vi "Copy InstrumentStudio Template.vi"(8 "error in":errorcluster) -> (0 "error out":errorcluster)   [LabVIEW 2021, in "Converter.lvlib"]
uses:
  Converter.lvlib
  Path Functions/Path Functions.lvlib
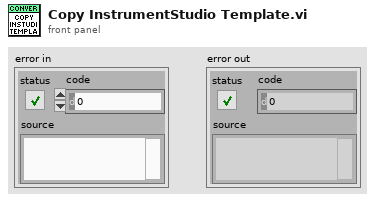
[diagram p1: front panel]
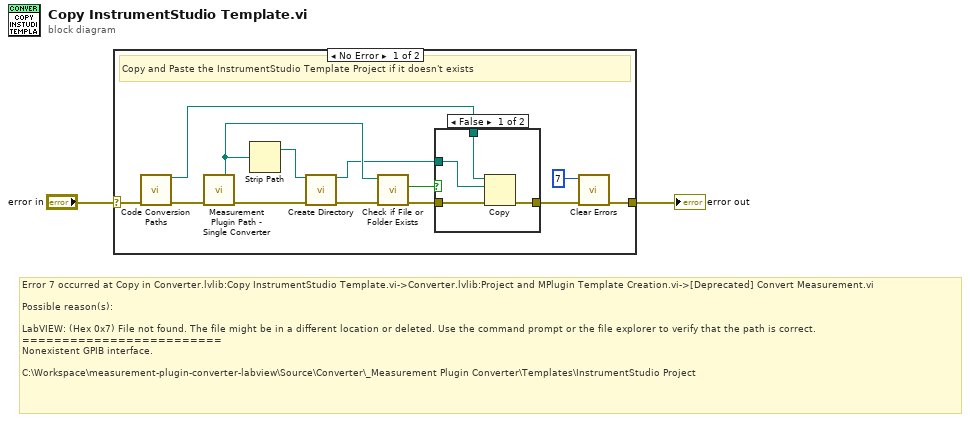
[diagram p0: block diagram]
diagram:
  # "Error 7 occurred at Copy in Converter.lvlib:Copy InstrumentStudio Template.vi->Converter.lvlib:Project and MPlugin Template Creation.vi->[Deprecated] Convert Measurement.vi\n\nPossible reason(s):\n\nLabVIEW: (Hex 0x7) File not found. The file might be in a different location or deleted. Use the command prompt or the file explorer to verify that the path is correct.\n=========================\nNonexistent GPIB interface.\n\nC:\\Workspace\\measurement-plugin-converter-labview\\Source\\Converter\\_Measurement Plugin Converter\\Templates\\InstrumentStudio Project"
  n1 = case shown="No Error" "error in" {
    selector: "error in" -> [w6 w21]
    tunnel: [w7 w21] -> w1
    frame No Error {
      # "Copy and Paste the InstrumentStudio Template Project if it doesn't exists"
      n2 = call "Code Conversion Paths.vi"("error in"=w6) -> ("is project directory"=w4:path, "error out"=w5:errorcluster)  [unwired: 6 in, 7 out]
      n3 = call "Measurement Plugin Path - Single Converter.vi"("error in"=w5) -> ("instrumentstudio folder"=w14:path, "error out"=w10:errorcluster)  [unwired: 2 in, 11 out]
      n4 = Strip Path(path=w14) -> (stripped path=w12:path)  [unwired: 1 out]
      n5 = call "Create Directory.vi"("directory"=w12, "error in"=w10) -> ("dup directory"=w11:path, "error out"=w9:errorcluster)  [unwired: 12 in]
      n6 = call <vilib>:"Check if File or Folder Exists.vi"("error in (no error)"=w9, "path"=w14) -> ("error out"=w8:errorcluster, "file or folder exists?"=w13:bool)  [unwired: 7 in, 1 out]
      n7 = case shown="False" w13 {
        tunnel: [w19 w20] -> w15
        tunnel: w4 -> [w18 _]
        tunnel: w11 -> [w17 _]
        tunnel: w8 -> [w16 w20]
        frame False {
          n8 = Copy(8:w16, 10:w17, 11:w18) -> (0:w19:errorcluster)  [unwired: 4 out]
        }
        frame True {
        }
      }
      n9 = call <vilib>:"Clear Errors.vi"("error in (no error)"=w15, "specific error code to clear (0: all)"=7) -> ("error out"=w7:errorcluster)  [unwired: 4 in, 1 out]
    }
    frame Error {
    }
  }
  "error out" <- w1
